vi "FWHM XDisplay.vi"(1 "calibration":dbl=1.0, 2 "array":dbl[](array[numeric])) -> (0 "FHWM":dbl)   [LabVIEW 2009, in "POLARIS IMAQ Display.xctl"]
uses:
  POLARIS IMAQ Display.xctl
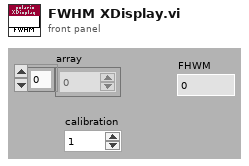
[diagram p1: front panel]
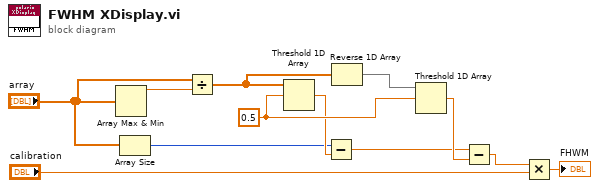
[diagram p0: block diagram]
diagram:
  w10 = 0.5 ("element")
  n1 = Array Max & Min(array="array") -> (max value=w12:dbl)  [unwired: 3 out]
  n2 = Array Size(array="array") -> (size(s)=w2:i32)
  n3 = Divide(x="array", y=w12) -> (x/y=w11:dbl[])
  n4 = Threshold 1D Array(2:w10, 3:w11) -> (0:w3:dbl)  [unwired: 1 in]
  n5 = Subtract(x=w2, y=w3) -> (x-y=w1:dbl)
  n6 = Reverse 1D Array(array=w11) -> (reversed array=w5:dbl[])
  n7 = Threshold 1D Array(2:w10, 3:w5) -> (0:w9:dbl)  [unwired: 1 in]
  n8 = Subtract(x=w1, y=w9) -> (x-y=w7:dbl)
  n9 = Multiply(x=w7, y="calibration") -> (x*y=→"FHWM":dbl)
